vi "String_to_Pathname.vi"(1 "Input String":string) -> (0 "path":path)   [LabVIEW 2010]
uses:
  Globals/Preference_global.vi
  Globals/Constants_global.vi
panel:
  out "size(s)":i32
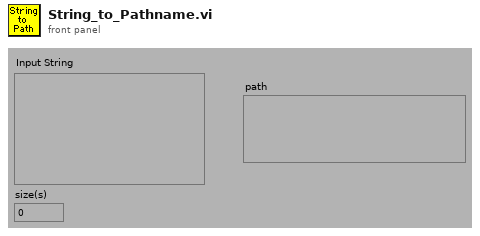
[diagram p1: front panel]
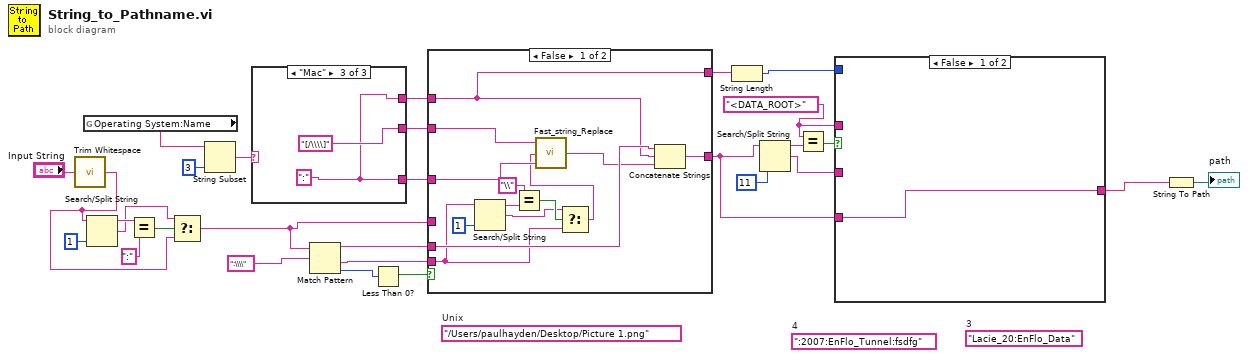
[diagram p0: block diagram]
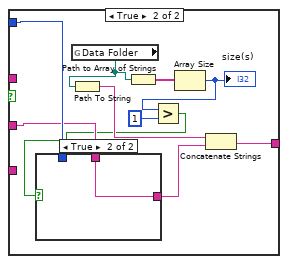
[diagram p2: hidden frame]
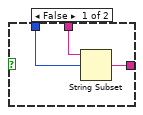
[diagram p3: hidden frame]
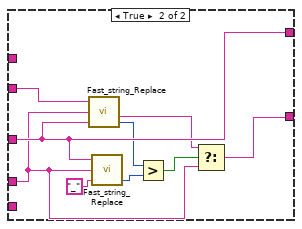
[diagram p4: hidden frame]
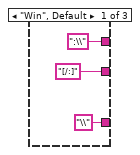
[diagram p5: hidden frame]
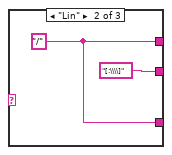
[diagram p6: hidden frame]
diagram:
  (unwired) "Lacie_20:EnFlo_Data"  # 3
  (unwired) ":2007:EnFlo_Tunnel:fsdfg"  # 4
  (unwired) "/Users/paulhayden/Desktop/Picture 1.png"  # Unix
  w8 = "<DATA_ROOT>" ("regular expression")
  n1 = call <vilib>:"Trim Whitespace.vi"("string"="Input String") -> ("trimmed string"=w1:string)  [unwired: 1 in]
  n2 = global read "Preference_global.vi" "Operating System:Name"() -> (w28:string)
  n3 = Search/Split String(string=w1, offset (0)=1 ("length (rest)")) -> (substring before match=w18:string, match + rest of string=w17:string)  [unwired: 2 out]
  n4 = Equal?(x=w18, y=":") -> (x = y?=w20:bool)
  n5 = Select(t=w17, s=w20, f=w1) -> (s? t:f=w16:string)
  n6 = String Subset(string=w28, length (rest)=3 ("length (rest)")) -> (substring=w29:string)  [unwired: 1 out]
  n7 = case shown="\"Mac\"" w29 {
    tunnel: ["[/:]" "[:\\\\]" "[/\\\\]"] -> w23
    tunnel: ["\\" w33 w35] -> w22
    tunnel: [":\\" w33 w35] -> w6
    frame "Win", Default {
    }
    frame "Lin" {
      w33 = "/"
    }
    frame "Mac" {
      w35 = ":"
    }
  }
  n8 = Match Pattern(string=w16, regular expression=":\\\\") -> (before substring=w14:string, after substring=w15:string, offset past match=w25:i32)  [unwired: 2 out]
  n9 = Less Than 0?(x=w25) -> (x < 0?=w24:bool)
  n10 = case shown="False" w24 {
    tunnel: w16 -> [_ w51]
    tunnel: w23 -> [w49 w58]
    tunnel: w22 -> [w48 w57]
    tunnel: w15 -> [w38 _]
    tunnel: w14 -> [w47 _]
    tunnel: w6 -> [w44 _]
    tunnel: [w45 w50] -> w11
    tunnel: [w44 w57] -> w3
    frame False {
      n11 = Search/Split String(string=w38, offset (0)=1 ("length (rest)")) -> (substring before match=w42:string, match + rest of string=w39:string)  [unwired: 2 out]
      n12 = Equal?(x="\\", y=w42) -> (x = y?=w40:bool)
      n13 = Select(t=w39, s=w40, f=w38) -> (s? t:f=w37:string)
      n14 = call "Fast_string_Replace.vi"("Replace match with:"=w48, "Input String"=w37, "regular expression"=w49) -> ("Output String"=w46:string)  [unwired: 2 out]
      n15 = Concatenate Strings(w47, w44, w46) -> (w45:string)
    }
    frame True {
      n16 = call "Fast_string_Replace.vi"("Replace match with:"=w57, "Input String"=w51, "regular expression"=w58) -> ("Number Found"=w55:i32, "Output String"=w52:string)  [unwired: 1 out]
      n17 = call "Fast_string_Replace.vi"("Replace match with:"="_", "Input String"=w51, "regular expression"=w57) -> ("Number Found"=w54:i32)  [unwired: 2 out]
      n18 = Greater?(x=w55, y=w54) -> (0:w53:bool)
      n19 = Select(t=w52, s=w53, f=w51) -> (s? t:f=w50:string)
    }
  }
  n20 = String Length(string=w3) -> (length=w4:i32)
  n21 = Search/Split String(string=w11, offset (0)=11) -> (substring before match=w13:string, match + rest of string=w7:string)  [unwired: 1 in, 1 out]
  n22 = Equal?(x=w8, y=w13) -> (x = y?=w12:bool)
  n23 = case shown="False" w12 {
    tunnel: w11 -> [w59 _]
    tunnel: [w59 w63] -> w10
    tunnel: w8 -> [_ _]
    tunnel: w7 -> [_ w67]
    tunnel: w4 -> [_ w68]
    frame False {
    }
    frame True {
      n24 = global read "Constants_global.vi" "Data Folder"() -> (w65:path)
      n25 = Path To String(path=w65) -> (string=w69:string)
      n26 = Path to Array of Strings(0:w65) -> (2:w64:string[])  [unwired: 1 out]
      n27 = Array Size(array=w64) -> (size(s)=w62:i32)
      "size(s)" <- w62
      n28 = Greater?(x=w62, y=1) -> (0:w60:bool)
      n29 = case shown="True" w60 {
        tunnel: w68 -> [w72 _]
        tunnel: w67 -> [w71 w73]
        tunnel: [w70 w73] -> w66
        frame False {
          n30 = String Subset(string=w71, offset (0)=w72) -> (substring=w70:string)  [unwired: 1 out]
        }
        frame True {
        }
      }
      n31 = Concatenate Strings(w69, w66) -> (w63:string)
    }
  }
  n32 = String To Path(string=w10) -> (path=→"path":path)
